vi "EnergyToXY.vi"() -> ()   [LabVIEW 2013]
panel:
  out "Array 3":dbl[](array[numeric])
  out "Array 2":dbl[](array[numeric])
  out "Array":dbl[](array[numeric])
  in  "FinalEnergy":dbl
  in  "InitalEnergy":dbl
  in  "EnergyStep":dbl
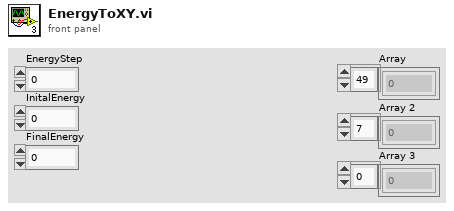
[diagram p1: front panel]
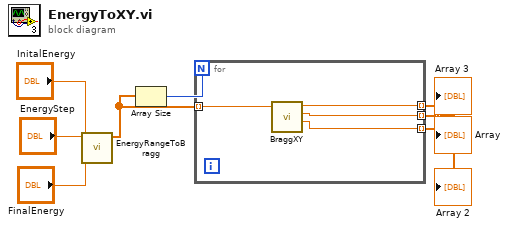
[diagram p0: block diagram]
diagram:
  n1 = call "EnergyRangeToBragg.vi"("FinalEnergy"="FinalEnergy", "InitalEnergy"="InitalEnergy", "EnergyStep"="EnergyStep") -> ("BraggArray"=w4:dbl[])  [unwired: 8 in]
  n2 = Array Size(array=w4) -> (size(s)=w5:i32)
  n3 = for {
    N: w5 -> [_]
    tunnel: w4 -> [w12] mode=indexing
    tunnel: [w11] -> w3 mode=indexing
    tunnel: [w10] -> w2 mode=indexing
    tunnel: [w9] -> w1 mode=indexing
    n4 = call "BraggXY.vi"("BraggAngle"=w12) -> ("YDesr"=w9:dbl, "XDest"=w10:dbl, "BraggAngle"=w11:dbl)  [unwired: 8 in]
  }
  "Array" <- w3
  "Array 2" <- w2
  "Array 3" <- w1
